vi "to_string.vi"(8 "error in (no error)":errorcluster, 11 "Table in":refnum<class "Table.lvclass">) -> (0 "error out":errorcluster, 1 "toml":string, 3 "Table out":refnum<class "Table.lvclass">)   [LabVIEW 2020, in "toml_edit.lvlib" / "Table.lvclass"]
uses:
  Table.lvclass
  Table.lvclass/Table.ctl
  toml_edit.lvlib
  dragon_toml_64.dll
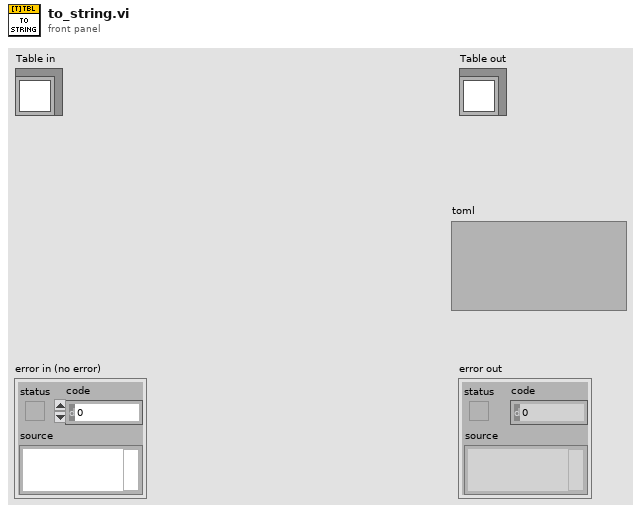
[diagram p1: front panel]
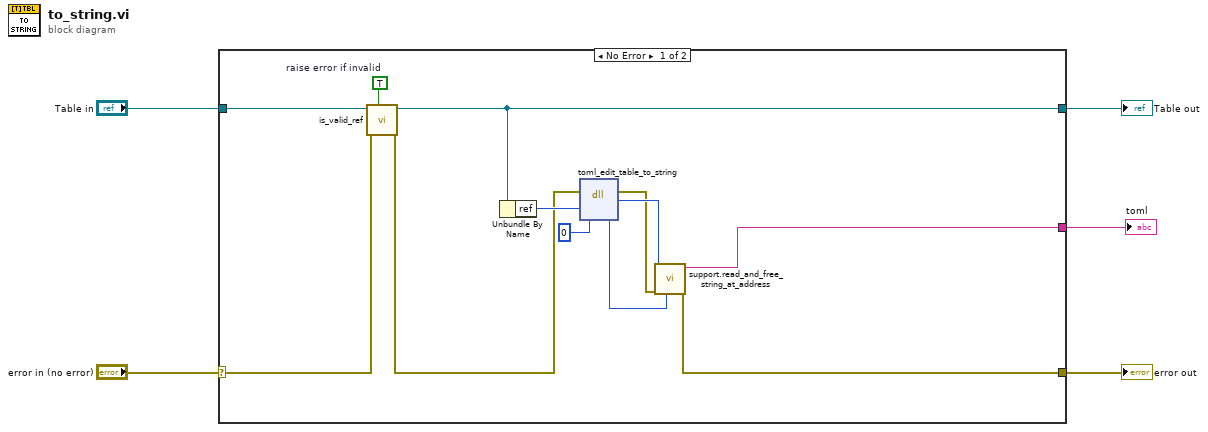
[diagram p0: block diagram]
diagram:
  n1 = case shown="No Error" "error in (no error)" {
    selector: "error in (no error)" -> [w9 w19]
    tunnel: [w13 w19] -> w4
    tunnel: [w11 w18] -> w2
    tunnel: "Table in" -> [w10 w18]
    tunnel: [w14 _] -> w1
    frame No Error {
      w12 = TRUE  # raise error if invalid
      n2 = call-dynamic "is_valid_ref.vi"("raise error if invalid? (False)"=w12, "error in (no error)"=w9, "Table in"=w10) -> ("error out"=w8:errorcluster, "Table out"=w11:refnum<class "Table.lvclass">)  [unwired: 6 in, 1 out]
      n3 = Unbundle By Name(w11) -> ("ref"=w15:u64)
      n4 = dll-call lib="C:/projects/dragon-desktop/source/submodules/toml-edit-labview/lv_src/dragon_toml_*.dll" fn="toml_edit_table_to_string"(error in=w8, "table_ref"=w15, "string_length"=u32 0) -> (error out=w16:errorcluster, "string_ptr"=w17:u64, "string_length"=w7:u32)  [unwired: 3 in, 1 out]
      n5 = call "support.read_and_free_string_at_address.vi"("string_length"=w7, "error in (no error)"=w16, "string_ptr"=w17) -> ("error out"=w13:errorcluster, "string"=w14:string)  [unwired: 7 in]
    }
    frame Error {
    }
  }
  "error out" <- w4
  "Table out" <- w2
  "toml" <- w1
